vi "Sub-Indices Count.vi"(11 "OD Entry in":refnum<class "OD Entry.lvclass">) -> (2 "size":i32, 3 "OD Entry out":refnum<class "OD Entry.lvclass">)   [LabVIEW 2024]
doc: "Number of Sub-Indices present in the object"
uses:
  OD Entry.lvclass/OD Entry.ctl
  OD Entry.lvclass
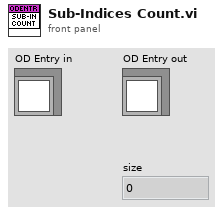
[diagram p1: front panel]
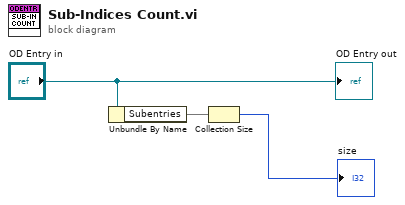
[diagram p0: block diagram]
diagram:
  n1 = Unbundle By Name("OD Entry in") -> ("Subentries"=w2)
  n2 = Collection Size(1:w2) -> (0:→"size":i32)
  "OD Entry out" <- "OD Entry in"
